vi "Read bomb status.vi"(8 "error in (no error)":errorcluster, 11 "RoomWithABomb in":refnum<class "RoomWithABomb.lvclass">) -> (0 "error out":errorcluster, 2 "bomb status":enum16{"none", "exploded", "unexploded"}(ring), 3 "RoomWithABomb out":refnum<class "RoomWithABomb.lvclass">)   [LabVIEW 2016, in "RoomWithABomb.lvclass"]
uses:
  RoomWithABomb.lvclass
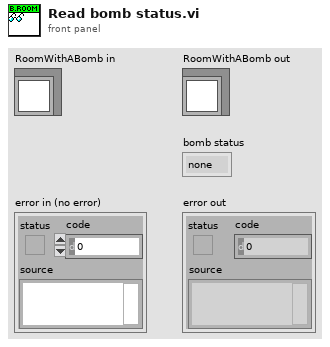
[diagram p1: front panel]
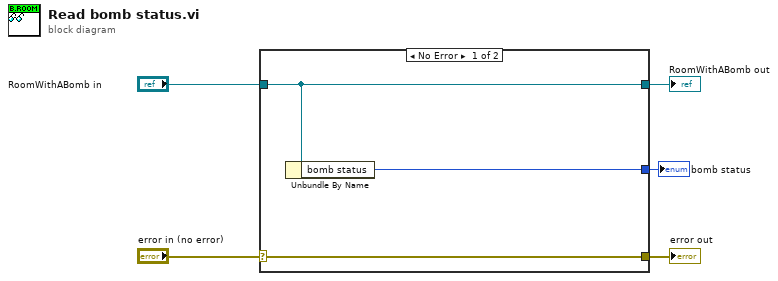
[diagram p0: block diagram]
diagram:
  n1 = case shown="No Error" "error in (no error)" {
    selector: "error in (no error)" -> [w8 w9]
    tunnel: [w8 w9] -> w4
    tunnel: [w7 w10] -> w2
    tunnel: "RoomWithABomb in" -> [w7 w10]
    tunnel: [w6 _] -> w1
    frame No Error {
      n2 = Unbundle By Name(w7) -> ("bomb status"=w6:enum16{"none", "exploded", "unexploded"})
    }
    frame Error {
    }
  }
  "error out" <- w4
  "RoomWithABomb out" <- w2
  "bomb status" <- w1
